vi "populateEventSettingsApplied.vi"(8 "error in (no error)":errorcluster, 10 "SettingsApplied":string, 11 "Model in":refnum<class "Model.lvclass">) -> (0 "error out":errorcluster, 3 "Model out":refnum<class "Model.lvclass">)   [LabVIEW 2016, in "Model.lvclass"]
uses:
  Model.lvclass
  Model.lvclass/Model.ctl
  Publisher/Publisher.lvclass/Publisher.ctl
  Publisher/Publisher.lvclass
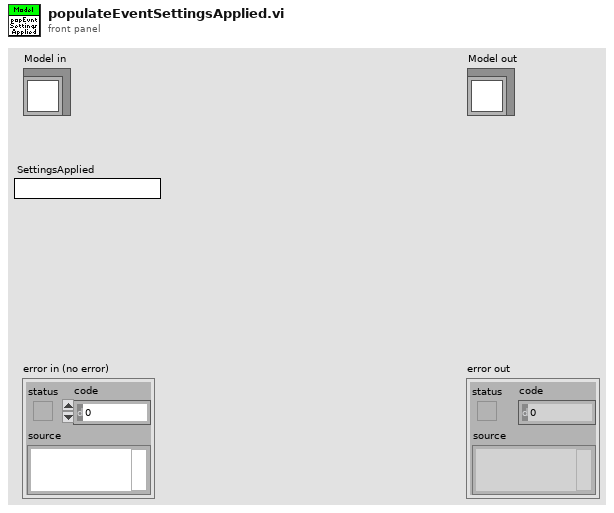
[diagram p1: front panel]
types:
  T1 = typedef "M1M3SupportTopics.lvlib/Timestamp.ctl" = dbl
  T2 = typedef "M1M3SupportTopics.lvlib/EventSettingsApplied.ctl" = cluster{"Timestamp":T1, "Settings":string}
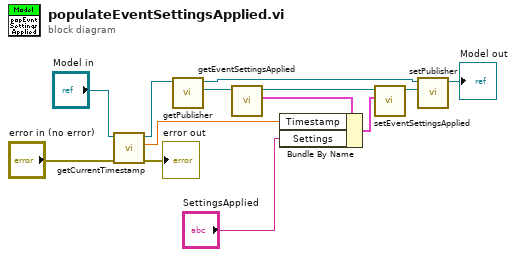
[diagram p0: block diagram]
diagram:
  n1 = call "getCurrentTimestamp.vi"("error in (no error)"="error in (no error)", "Model in"="Model in") -> ("error out"=→"error out":errorcluster, "Timestamp"=w6:T1, "Model out"=w13:refnum<class "Model.lvclass">)  [unwired: 7 in]
  n2 = call "getPublisher.vi"("Model in"=w13) -> ("Publisher"=w10:refnum<class "Publisher.lvclass">, "Model out"=w12:refnum<class "Model.lvclass">)  [unwired: 9 in]
  n3 = call "getEventSettingsApplied.vi"("Publisher in"=w10) -> ("EventSettingsApplied"=w7:T2, "Publisher out"=w9:refnum<class "Publisher.lvclass">)  [unwired: 9 in]
  n4 = Bundle By Name(cluster=w7, "Timestamp"=w6, "Settings"="SettingsApplied") -> (w5:T2)
  n5 = call "setEventSettingsApplied.vi"("EventSettingsApplied"=w5, "Publisher in"=w9) -> ("Publisher out"=w8:refnum<class "Publisher.lvclass">)  [unwired: 9 in]
  n6 = call "setPublisher.vi"("Publisher"=w8, "Model in"=w12) -> ("Model out"=→"Model out":refnum<class "Model.lvclass">)  [unwired: 9 in]
